vi "Calculate Peak.vi"(8 "error in":errorcluster, 10 "Function":string(combo), 11 "VISA resource name in":refnum<visa-resource-name>) -> (0 "error out":errorcluster, 2 "Value":dbl, 3 "VISA resource name out":refnum<visa-resource-name>)   [LabVIEW 2021, in "Keysight U1282A.lvlib"]
doc: "El comando de calcular pico ( CALC:PEAK) regresa el valor de la función peak-hold:\n-Maximum - regresa el máximo valor registrado.\n-Minimum - regresa el mínimo valor registrado."
uses:
  Keysight U1282A.lvlib
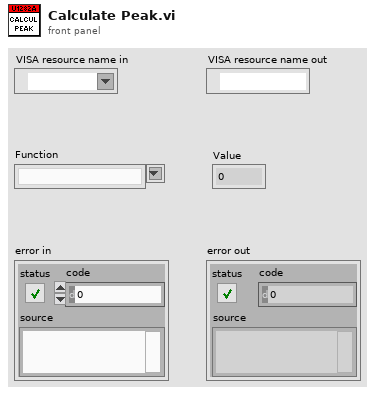
[diagram p1: front panel]
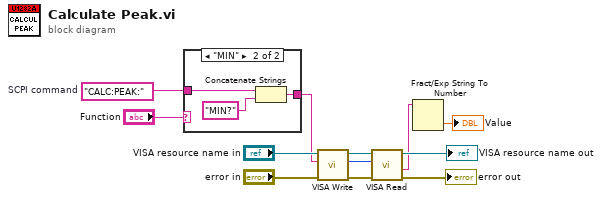
[diagram p0: block diagram]
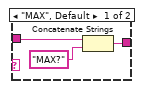
[diagram p2: hidden frame]
diagram:
  w4 = "CALC:PEAK:"  # SCPI command
  n1 = case shown="\"MIN\"" "Function" {
    tunnel: w4 -> [w14 w17]
    tunnel: [w13 w16] -> w3
    frame "MAX", Default {
      n2 = Concatenate Strings(w14, "MAX?") -> (w13:string)
    }
    frame "MIN" {
      n3 = Concatenate Strings(w17, "MIN?") -> (w16:string)
    }
  }
  n4 = call "VISA Write.vi"("error in"="error in", "SCPI command"=w3, "VISA resource in"="VISA resource name in") -> ("error out"=w12:errorcluster, "Bytes at Port out"=w10:u32, "VISA resource out"=w11:refnum<visa-resource-name>)  [unwired: 6 in]
  n5 = call "VISA Read.vi"("error in"=w12, "Bytes at Port in"=w10, "VISA resource in"=w11) -> ("error out"=→"error out":errorcluster, "Reading"=w1:string, "VISA resource out"=→"VISA resource name out":refnum<visa-resource-name>)  [unwired: 5 in, 1 out]
  n6 = Fract/Exp String To Number(string=w1) -> (number=→"Value":dbl)  [unwired: 3 in, 1 out]
